vi "Keithley 27XX Data Information.vi"() -> ()   [LabVIEW 2020]
doc: "This example VI shows how to use the Data Elements Selector to show more information about the data."
uses:
  <instrlib>/Keithley 27XX/Public/Data/Read Multiple Direct.vi
  <instrlib>/Keithley 27XX/Keithley 27XX.lvlib
panel:
  in  "Serial Configuration":T1={"Baud Rate (9600)"=9600, "Flow Control (1: XON/XOFF)"=1, "Termination Char (0:CR)"=0} {"Termination Char (0:CR)" items=["CR", "LF", "CRLF (Do not use)", "LFCR (Do not use)"]; "Flow Control (1: XON/XOFF)" items=["None", "XON/XOFF", "RTS/CTS (2701 Only)", "XON/XOFF & RTS/CTS (2701 Only)"]; "Baud Rate (9600)" items=["300"=300, "600"=600, "1200"=1200, "2400"=2400, "4800"=4800, "9600"=9600, "19.2k"=19200, "38.4k (2701 Only)"=38400, "57.6k (2701 Only)"=57600, "115.2k (2701 Only)"=115200]}
  in  "Timeout (30000 milliseconds)":u32=30000
  out "Channel":string[](array[string])
  out "Measurement Data":dbl[](array[numeric])
  out "Timestamp":string[](array[string])
  in  "Function (0: DC Voltage)":u16(ring) items=["DC Voltage", "AC Voltage", "DC Current", "AC Current", "Resistance", "Four-Wire Resistance", "Temperature (C)", "Frequency", "Period", "Continuity"]
  in  "Sample Count (10)":i32=10
  in  "Channel List (101:110)":string="101:110"
  in  "VISA resource name":refnum<visa-resource-name>
  # "© 2005 National Instruments Corporation.  ALL RIGHTS RESERVED."
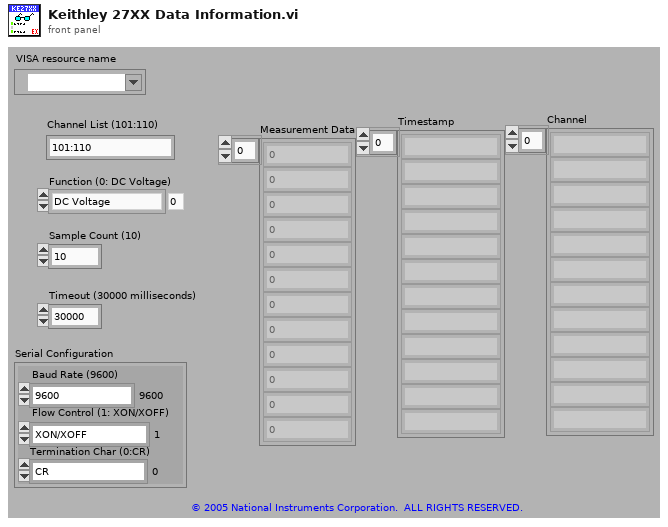
[diagram p1: front panel]
types:
  T1 = cluster{"Baud Rate (9600)":u32, "Flow Control (1: XON/XOFF)":u16, "Termination Char (0:CR)":u16}
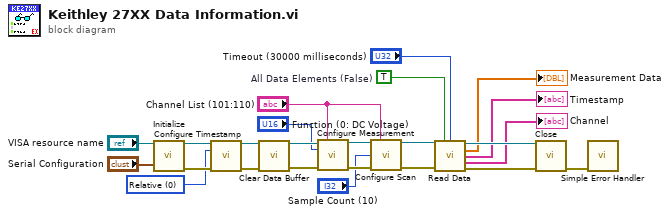
[diagram p0: block diagram]
diagram:
  w3 = TRUE  # All Data Elements (False)
  w8 = u16 0 items=["Relative", "Real Time Clock"] ("Timestamp Type (0: Relative)")
  n1 = call <instrlib>:"Initialize.vi"("VISA resource name"="VISA resource name", "Serial Configuration"="Serial Configuration") -> ("VISA resource name out"=w9:refnum<visa-resource-name>, "error out"=w10:errorcluster)  [unwired: 12 in]
  n2 = call <instrlib>:"Configure Timestamp.vi"("VISA resource name"=w9, "Timestamp Type (0: Relative)"=w8, "error in (no error)"=w10) -> ("VISA resource name out"=w12:refnum<visa-resource-name>, "error out"=w11:errorcluster)  [unwired: 11 in]
  n3 = call <instrlib>:"Clear Data Buffer.vi"("VISA resource name"=w12, "error in (no error)"=w11) -> ("VISA resource name out"=w5:refnum<visa-resource-name>, "error out"=w16:errorcluster)  [unwired: 12 in]
  n4 = call <instrlib>:"Configure Measurement.vi"("VISA resource name"=w5, "Scan List (Empty)"="Channel List (101:110)", "Function (0: DC Voltage)"="Function (0: DC Voltage)", "error in (no error)"=w16) -> ("VISA resource name out"=w23:refnum<visa-resource-name>, "error out"=w19:errorcluster)  [unwired: 10 in]
  n5 = call <instrlib>:"Configure Scan.vi"("VISA resource name"=w23, "Channel List (101:110)"="Channel List (101:110)", "Sample Count (100)"="Sample Count (10)", "error in (no error)"=w19) -> ("VISA resource name out"=w14:refnum<visa-resource-name>, "error out"=w15:errorcluster)  [unwired: 10 in]
  n6 = call-poly <instrlib>:"Read Data.vi"("VISA resource name"=w14, "All Data Elements (False)"=w3, "Timeout (30000 milliseconds)"="Timeout (30000 milliseconds)", "error in (no error)"=w15) -> ("VISA resource name out"=w22:refnum<visa-resource-name>, "Measurement Data"=→"Measurement Data":dbl[], "Time Stamp"=→"Timestamp":string[], "Channel"=→"Channel":string[], "error out"=w21:errorcluster)  [unwired: 6 in, 1 out]
  n7 = call <instrlib>:"Close.vi"("VISA resource name"=w22, "error in (no error)"=w21) -> ("error out"=w18:errorcluster)  [unwired: 13 in]
  n8 = call <vilib>:"Simple Error Handler.vi"("error in (no error)"=w18) -> ()  [unwired: 4 in, 5 out]
